vi "produceTimingTicks.vi"(8 "error in (no error)":errorcluster, 10 "Channel":refnum<class "Channel.lvclass">, 11 "ScriptEventList in":refnum<class "ScriptEventList.lvclass">) -> (0 "error out":errorcluster, 2 "timingTickList":refnum<class "ScriptEventList.lvclass">, 3 "ScriptEventList out":refnum<class "ScriptEventList.lvclass">)   [LabVIEW 2011, in "Tools.lvlib" / "Scripting.lvlib" / "ScriptEventList.lvclass"]
uses:
  ScriptEventList.lvclass
  DatabaseHelpers/Database Objects/Channel/Channel.lvclass
  ScriptEventList.lvclass/ScriptEventList.ctl
  ScriptEvent.lvclass
panel:
  out "Array 2":dbl[](array[numeric]) format="%_10g"
  out "Array":dbl[][](array[numeric]) format="%_10g"
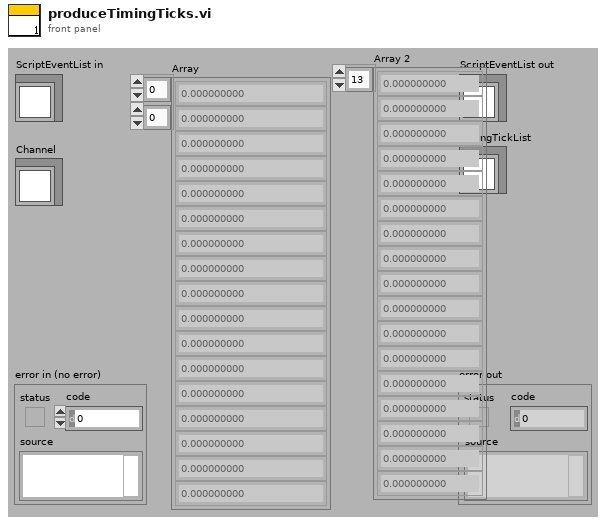
[diagram p1: front panel]
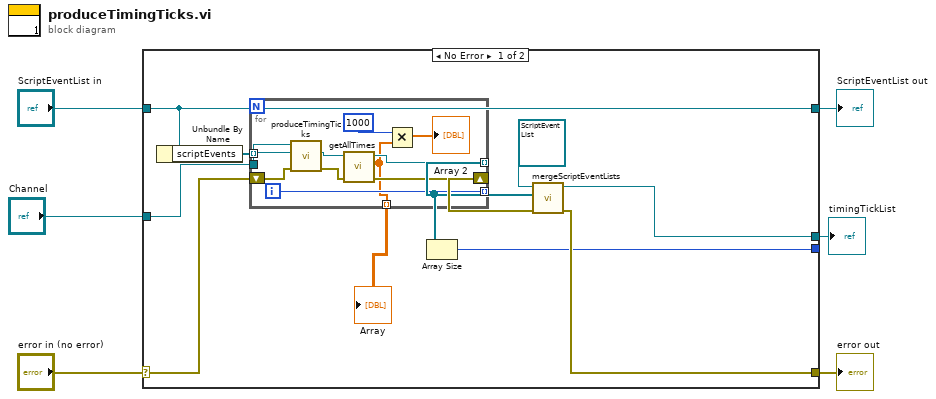
[diagram p0: block diagram]
diagram:
  n1 = case shown="No Error" "error in (no error)" {
    selector: "error in (no error)" -> [w15 w29]
    tunnel: [w10 w29] -> w5
    tunnel: [w17 w28] -> w3
    tunnel: "ScriptEventList in" -> [w17 w28]
    tunnel: [w12 _] -> w2
    tunnel: "Channel" -> [w14 _]
    tunnel: [w8 _] -> _
    frame No Error {
      n2 = Unbundle By Name(w17) -> ("scriptEvents"=w16:refnum<class "ScriptEvent.lvclass">[])
      n3 = for {
        tunnel: w16 -> [w27] mode=indexing
        shift-right: [w25] -> w11
        shift-left: w15 -> [w26]
        tunnel: [w21] -> w9 mode=indexing
        tunnel: w14 -> [w24]
        tunnel: [w23] -> _ mode=indexing
        tunnel: [w20] -> w7 mode=indexing
        i -> [w23]
        n4 = call-dynamic "produceTimingTicks.vi"("error in (no error)"=w26, "Channel"=w24, "ScriptEvent in"=w27) -> ("error out"=w25:errorcluster, "timingTick"=w22:refnum<class "ScriptEventList.lvclass">)  [unwired: 6 in, 1 out]
        n5 = call "getAllTimes.vi"("ScriptEventList in"=w22) -> ("Array"=w20:dbl[], "ScriptEventList out"=w21:refnum<class "ScriptEventList.lvclass">)  [unwired: 8 in, 1 out]
        n6 = Multiply(x=1000, y=w20) -> (x*y=→"Array 2":dbl[])
      }
      "Array" <- w7
      n7 = Array Size(array=w9) -> (size(s)=w8:i32)
      n8 = call "mergeScriptEventLists.vi"("error in (no error)"=w11, "Array"=w9, "ScriptEventList in"=refnum<class "ScriptEventList.lvclass"> refnum) -> ("error out"=w10:errorcluster, "ScriptEventList out"=w12:refnum<class "ScriptEventList.lvclass">)  [unwired: 7 in]
    }
    frame Error {
    }
  }
  "error out" <- w5
  "ScriptEventList out" <- w3
  "timingTickList" <- w2
